vi "Hide Cursor.vi"(0 "Show(T, default) or Hide(F) Cursor":bool=TRUE) -> ()   [LabVIEW 2011]
doc: "This example will Hide or Show the cursor when inside a LabVIEW window. This VI basically calls the ShowCursor function in User32.dll. \n\nNote: While the cursor is hidden, it is still there, i.e. you can still move it and click on an object, even though you can't see the cursor."
uses:
  user32.dll
panel:
  # "This example will Hide or Show the cursor when inside a LabVIEW \nwindow.  This VI basically calls the ShowCursor function in User32.dll.  \n\nNote:  While the cursor is hidden, it is still there, i.e. you can still move \n             it and click on an object, even though you can't see the cursor."
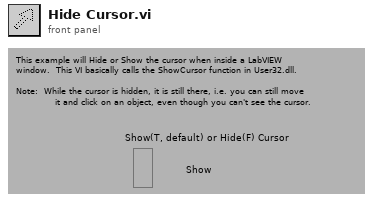
[diagram p1: front panel]
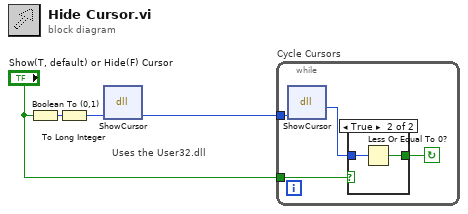
[diagram p0: block diagram]
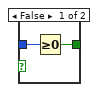
[diagram p2: hidden frame]
diagram:
  # "Uses the User32.dll"
  n1 = Boolean To (0,1)(Boolean="Show(T, default) or Hide(F) Cursor") -> (0, 1=w4:i16)
  n2 = To Long Integer(number=w4) -> (32bit integer=w2:i32)
  n3 = dll-call lib="User32.dll" fn="ShowCursor" label="int16 ShowCursor(int32 Enable);"("Enable"=w2) -> ("Enable"=w3:i32)  [unwired: 3 in, 3 out]
  n4 = while "Cycle Cursors" {
    tunnel: "Show(T, default) or Hide(F) Cursor" -> [w5]
    tunnel: w3 -> [w8]
    stop <- w6 continue-if-true
    n5 = dll-call lib="User32.dll" fn="ShowCursor" label="int16 ShowCursor(int32 Enable);"("Enable"=w8) -> (w7:i16)  [unwired: 4 in, 2 out]
    n6 = case shown="True" w5 {
      tunnel: w7 -> [w10 w12]
      tunnel: [w9 w11] -> w6
      frame False {
        n7 = Greater Or Equal To 0?(x=w10) -> (x >= 0?=w9:bool)
      }
      frame True {
        n8 = Less Or Equal To 0?(x=w12) -> (x <= 0?=w11:bool)
      }
    }
  }
